vi "CheckDeviceExptDefaultExpt.vi"(10 "Expt name / MCIP/ Variable/Preset Name":string) -> (2 "DevicesNotInExperiment":string[](array[string]))   [LabVIEW 2020]
uses:
  Shared/MySQL/Preset Query Enum.ctl
  <userlib>/_OpenG.lib/array/array.llb/Empty 2D Array (String)__ogtk.vi
panel:
  out "String":string
  out "Multicolumn Listbox":i32[](listbox)
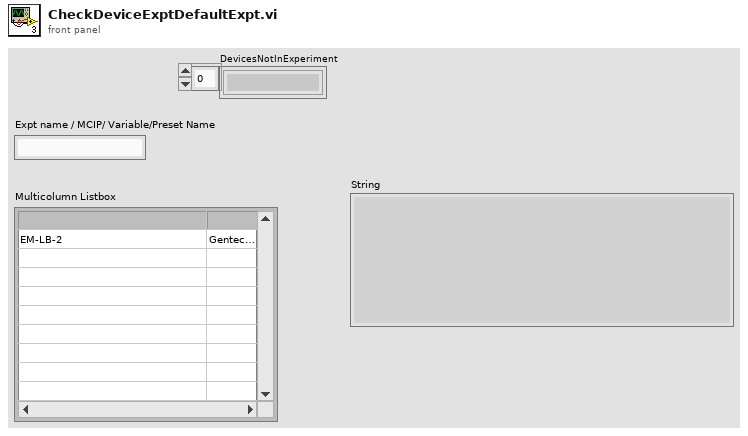
[diagram p1: front panel]
types:
  T1 = typedef "Preset Query Enum.ctl" = enum16{"Get Locations", "Get all IPs and MACs", "Get classes", "Get expt variables to set at scanstart for particular device", "Get expt devices and variables with start values", "Get expt devices and variables (with data to get)", "Get expt devices with data to get", "Get Expt devices and GUIs", "Get all devices basic properties", "Get Virtual Devices Core Info", "Get Expt names", "Get experiment basic properties", "Get experiment alarm variables", "Get MC Ports", "Get device network comm port", "Get devicetype lvclass path", "Get basic device properties", "Get Init Order", "Get all setable variables of a device", "Get device variable aliases", "Get force values of all settable variables", "Get all variables of a devicetype", "Get all variables of a device", "Get plotter details", "Get Saved Scans", "Get Scan Info", "GetGeneralGUIs", "Get expt for plotter", "Get plotter IDs from expt", "Get all devices", "Get all Virtual Devices", "Get all aliases", "Get variable and device info for Virtual Device", "GetItemLocatorIP", "Get IPs for GUIs", "Get DeviceType from Device", "GetLocalPortRange", "GetDevicePresetVariables", "Get Device Configuration", "GetAllPresetNames", "GetAllConfigurationNames", "GetPresetDeviceNames", "GetDeviceAliases", "GetDevicesOfClass"}
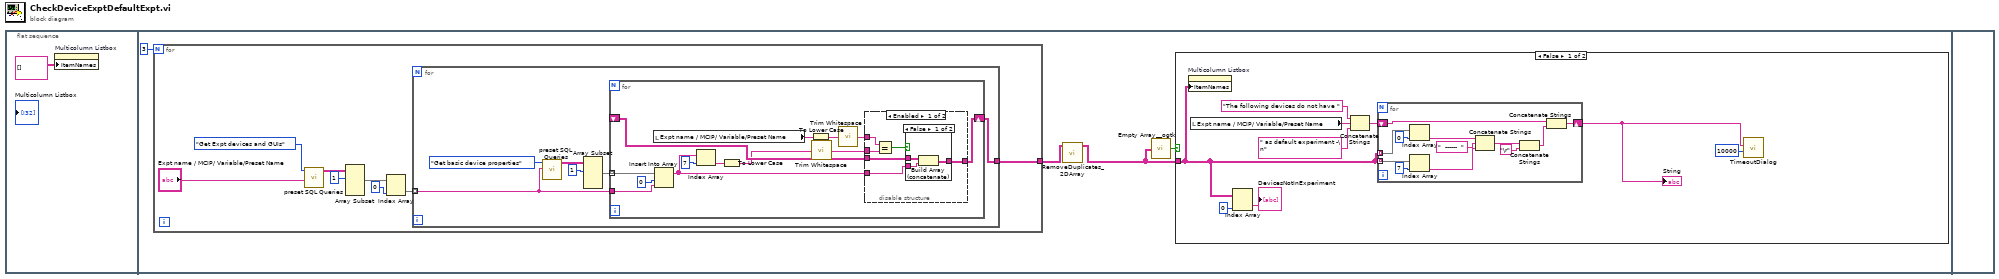
[diagram p0: block diagram]
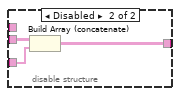
[diagram p3: hidden frame]
diagram:
  n1 = flat-sequence {
    frame #0 {
      n2 = property on="Multicolumn Listbox" class="MCListbox (strict)"("ItemNames"=string[][] [] ("Item Names")) -> ()  [unwired: 2 in, 2 out]
    }
    frame #1 {
      n3 = for {
        N: 3 -> [_]
        tunnel: [w6] -> w4
        n4 = call "preset SQL Queries.vi"("Expt name / MCIP/ Variable/Preset Name"="Expt name / MCIP/ Variable/Preset Name", "Preset Query"=Preset_Query_Enum."Get Expt devices and GUIs") -> ("data"=w11:string[][])  [unwired: 7 in, 2 out]
        n5 = Array Subset(array=w11, index (row)=1 ("disabled index (col)")) -> (w9:string[][])  [unwired: 3 in]
        n6 = Index Array(array=w9, index (col)=0 ("disabled index (col)")) -> (element=w7:string[])  [unwired: 1 in]
        n7 = for {
          tunnel: w7 -> [w18] mode=indexing
          tunnel: [w17] -> w6
          n8 = call "preset SQL Queries.vi"("Device/Devicetype name\n/Plotter.id/ScanName#"=w18, "Preset Query"=Preset_Query_Enum."Get basic device properties") -> ("data"=w16:string[][])  [unwired: 7 in, 2 out]
          n9 = Array Subset(array=w16, index (row)=1) -> (w14:string[][])  [unwired: 3 in]
          n10 = for {
            tunnel: w18 -> [w32]
            shift-right: [w30] -> w17
            shift-left: _ -> [w29]
            tunnel: w14 -> [w28] mode=indexing
            n11 = local read "Expt name / MCIP/ Variable/Preset Name"() -> (w25:string)
            n12 = Insert Into Array(array=w28, index=0, new element=w32) -> (w27:string[])
            n13 = Index Array(array=w27, index=7) -> (element=w24:string)
            n14 = To Lower Case(string=w24) -> (all lower case string=w23:string)
            n15 = To Lower Case(string=w25) -> (all lower case string=w21:string)
            n16 = call <vilib>:"Trim Whitespace.vi"("string"=w23) -> ("trimmed string"=w22:string)  [unwired: 1 in]
            n17 = call <vilib>:"Trim Whitespace.vi"("string"=w21) -> ("trimmed string"=w20:string)  [unwired: 1 in]
            n18 = disable-structure shown="Enabled" {
              disable-tunnel: [w38 w43] -> w30
              disable-tunnel: w29 -> [w37 w44]
              disable-tunnel: w27 -> [w36 w45]
              disable-tunnel: w22 -> [w35 _]
              disable-tunnel: w20 -> [w34 _]
              frame Enabled {
                n19 = Equal?(x=w34, y=w35) -> (x = y?=w33:bool)
                n20 = case shown="False" w33 {
                  tunnel: w36 -> [w41 _]
                  tunnel: [w40 w42] -> w38
                  tunnel: w37 -> [w39 w42]
                  frame False {
                    n21 = Build Array (concatenate)(w39, w41) -> (w40:string[][])
                  }
                  frame True {
                  }
                }
              }
              frame Disabled {
                n22 = Build Array (concatenate)(w44, w45) -> (w43:string[][])
              }
            }
          }
        }
      }
      n23 = call "RemoveDuplicates_2DArray.vi"("Input Array"=w4) -> ("Removed Duplicate Array"=w3:string[][])  [unwired: 10 in]
      n24 = call-poly <userlib>:"Empty Array__ogtk.vi"("Array"=w3) -> ("Empty Array?"=w5:bool)  [unwired: 8 in]
      n25 = case shown="False" w5 {
        tunnel: w3 -> [w48 _]
        frame False {
          n26 = property on="Multicolumn Listbox" class="MCListbox (strict)"("ItemNames"=w48) -> ()  [unwired: 2 in, 2 out]
          n27 = local read "Expt name / MCIP/ Variable/Preset Name"() -> (w54:string)
          n28 = Index Array(array=w48, index (col)=0 ("disabled index (col)")) -> (element=→"DevicesNotInExperiment":string[])  [unwired: 1 in]
          n29 = Concatenate Strings("The following devices do not have ", w54, " as default experiment -\n" ("string")) -> (w51:string)
          n30 = for {
            tunnel: w48 -> [w66] mode=indexing
            tunnel: w48 -> [w65] mode=indexing
            shift-right: [w59] -> w50
            shift-left: w51 -> [w58]
            n31 = Index Array(array=w66, index=0) -> (element=w61:string)
            n32 = Index Array(array=w65, index=7) -> (element=w62:string)
            n33 = Concatenate Strings(w61, "  ------  " ("string"), w62) -> (w56:string)
            n34 = Concatenate Strings(w56, "\r") -> (w55:string)
            n35 = Concatenate Strings(w58, w55) -> (w59:string)
          }
          "String" <- w50
          n36 = call "TimeoutDialog.vi"("message 2"=w50, "Timeout(ms)"=u32 10000) -> ()  [unwired: 9 in]
        }
        frame True {
        }
      }
    }
    frame #2 {
    }
  }
